vi "AssertsAlmostEqual.vi"(0 "VI Reference In":refnum<vi>, 1 "Label (VI Title)":string="Default", 11 "error in (no error)":errorcluster) -> (4 "VI Reference Out":refnum<vi>, 15 "error out":errorcluster)   [LabVIEW 2016, in "Drona Test.lvlib"]
uses:
  Drona Test.lvlib
  main/apis/Stimulus/KeyBoardSimulation/ValueSignalLatchBooleanString.vi
  main/apis/Assert/AssertControlValue/AlmostEqual.vi
  <vilib>/addons/_JKI Toolkits/Caraya/classes/Assert/Assert Not Error.vi
  <vilib>/addons/_JKI Toolkits/Caraya/classes/Assert/Assert Error.vi
  <vilib>/addons/_JKI Toolkits/Caraya/classes/Test/Test.lvclass
  main/Drona.lvlib
  <vilib>/addons/_JKI Toolkits/Caraya/classes/Assert/Assert.lvclass
  main/apis/Stimulus/KeyBoardSimulation/KeyboardSimulation.lvlib
  main/apis/Assert/AssertControlValue/AssertControlValue.lvlib
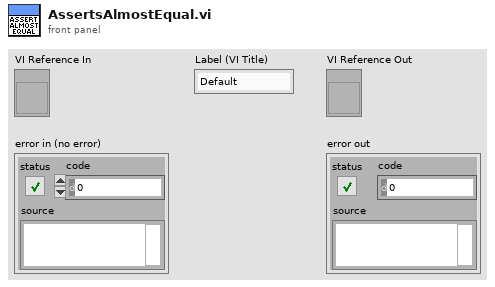
[diagram p1: front panel]
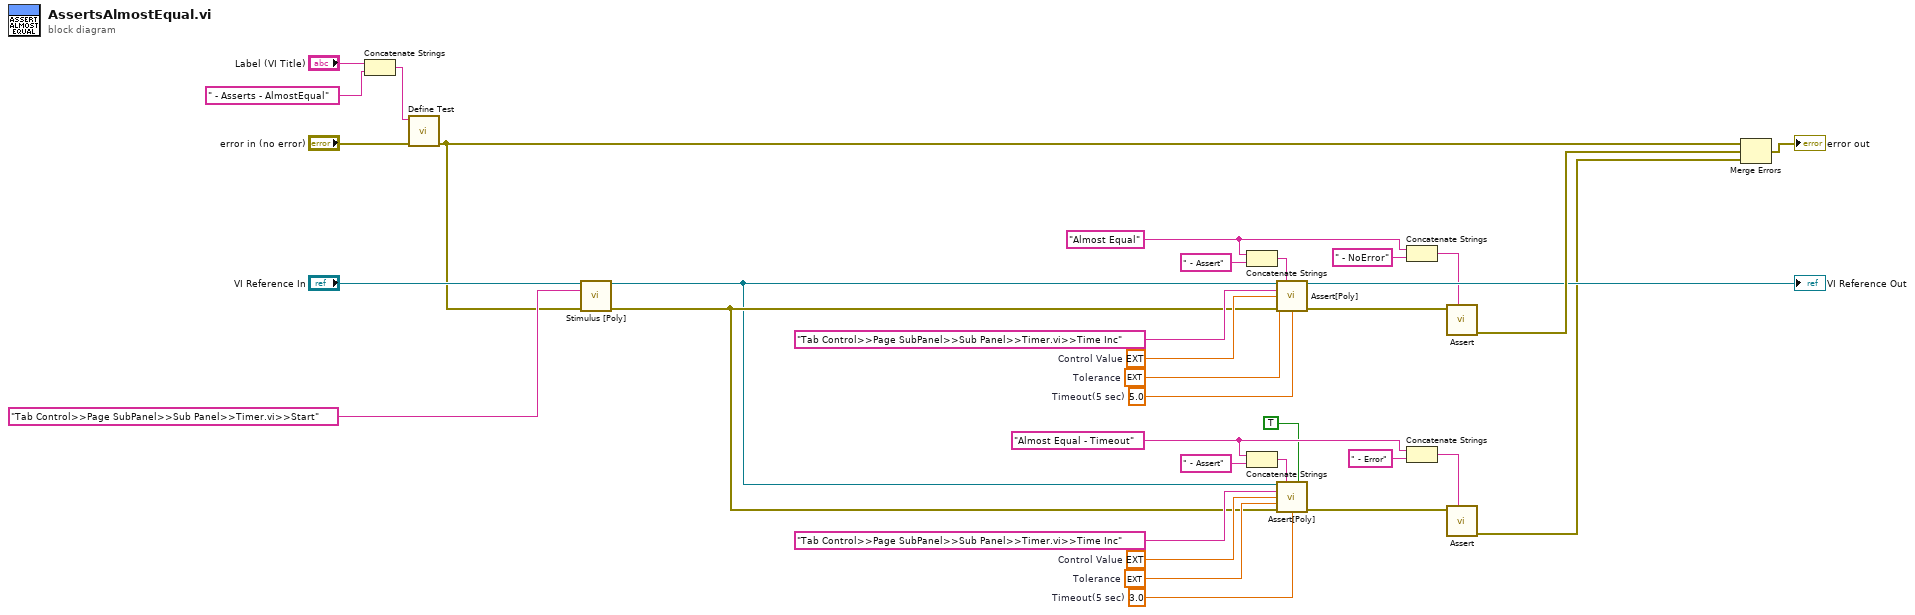
[diagram p0: block diagram]
diagram:
  w3 = ext 0.5  # Tolerance
  w4 = ext 0.5  # Tolerance
  w14 = 3.0  # Timeout(5 sec)
  w13 = ext 5.0  # Control Value
  w12 = "Almost Equal - Timeout" ("string")
  w15 = 5.0  # Timeout(5 sec)
  w16 = ext 5.0  # Control Value
  w17 = "Almost Equal" ("string")
  n1 = Concatenate Strings("Label (VI Title)", " - Asserts - AlmostEqual" ("Label (VI Title)")) -> (w29:string)
  n2 = call <vilib>:"Define Test.vi"("error in (no error)"="error in (no error)", "Label (VI Title)"=w29) -> ("error out"=w24:errorcluster)  [unwired: 9 in]
  n3 = call-poly "Stimulus [Poly].vi"("VI Reference In"="VI Reference In", "Control Path"="Tab Control>>Page SubPanel>>Sub Panel>>Timer.vi>>Start", "error in"=w24) -> ("VI Reference Out"=w1:refnum<vi>, "error out"=w2:errorcluster)  [unwired: 11 in]
  n4 = Concatenate Strings(w17, " - Assert" ("string")) -> (w19:string)
  n5 = Concatenate Strings(w12, " - Assert" ("string")) -> (w10:string)
  n6 = call-poly "Assert[Poly].vi"("VI Reference In"=w1, "Label"=w19, "Control Path"="Tab Control>>Page SubPanel>>Sub Panel>>Timer.vi>>Time Inc", "Control Value"=w16, "Tolerance"=w4, "Error In"=w2, "Timeout(5 sec)"=w15) -> ("VI Reference Out"=→"VI Reference Out":refnum<vi>, "Error Out"=w20:errorcluster)  [unwired: 7 in]
  n7 = call-poly "Assert[Poly].vi"("VI Reference In"=w1, "Label"=w10, "Assert Only? (F)"=TRUE, "Control Path"="Tab Control>>Page SubPanel>>Sub Panel>>Timer.vi>>Time Inc", "Control Value"=w13, "Tolerance"=w3, "Error In"=w2, "Timeout(5 sec)"=w14) -> ("Error Out"=w9:errorcluster)  [unwired: 6 in, 1 out]
  n8 = Concatenate Strings(w17, " - NoError" ("string")) -> (w18:string)
  n9 = Concatenate Strings(w12, " - Error" ("string")) -> (w11:string)
  n10 = call-poly <vilib>:"Assert.vi"("Label"=w18, "Not Error?"=w20) -> ("error out"=w34:errorcluster)  [unwired: 9 in]
  n11 = call-poly <vilib>:"Assert.vi"("Label"=w11, "Error?"=w9) -> ("error out"=w25:errorcluster)  [unwired: 9 in]
  n12 = Merge Errors(w24, w34, w25) -> (→"error out":errorcluster)
